vi "Send.vi"(8 "error in (no error)":errorcluster, 10 "Message":refnum<class "BaseMessage.lvclass">, 11 "QueueReader in":refnum<class "MultiQueueReader.lvclass">) -> (0 "error out":errorcluster, 2 "Sent Message":refnum<class "BaseMessage.lvclass">, 3 "QueueReader out":refnum<class "MultiQueueReader.lvclass">)   [LabVIEW 2025, in "MultiQueueReader.lvclass"]
doc: "Send a message to the remote destination"
uses:
  MultiQueueReader.lvclass
  Message/BaseMessage/BaseMessage.lvclass
  MultiQueueReader.lvclass/MultiQueueReader.ctl
  BaseReader/BaseReader.lvclass
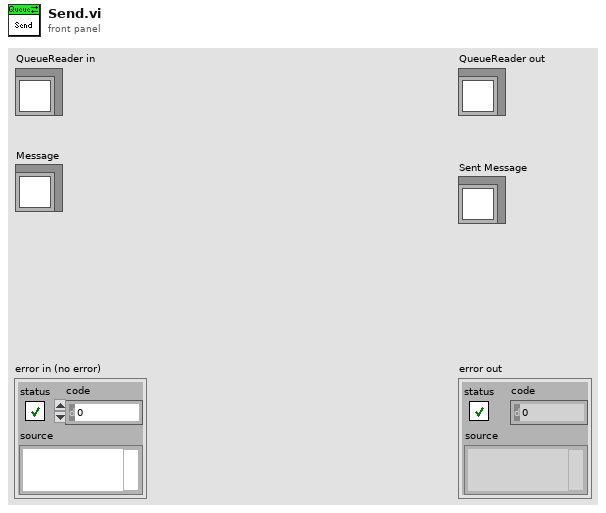
[diagram p1: front panel]
types:
  T1 = typedef "message_queue.ctl" = refnum<queue>
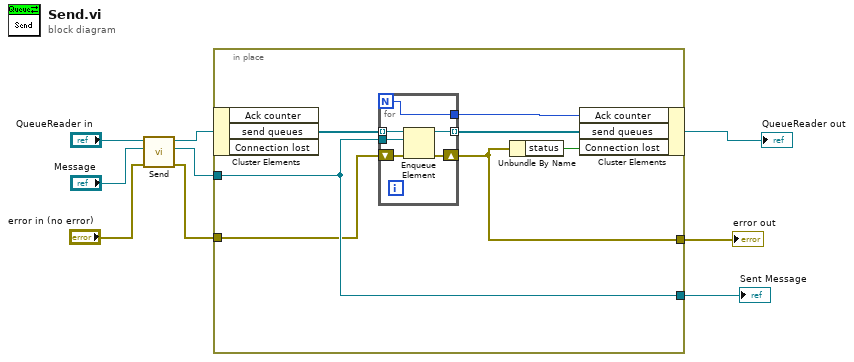
[diagram p0: block diagram]
diagram:
  n1 = call-parent "Send.vi"("error in (no error)"="error in (no error)", "Message"="Message", "BaseReader in"="QueueReader in") -> ("error out"=w1:errorcluster, "Sent Message"=w3:refnum<class "BaseMessage.lvclass">, "BaseReader out"=w5:refnum<class "MultiQueueReader.lvclass">)  [unwired: 6 in]
  n2 = in-place "In Place Element Structure" {
    in-place-border: w3 -> [w16]
    in-place-border: [w16] -> w9
    in-place-border: w1 -> [w14]
    in-place-border: [w12] -> w7
    n3 = in-place-cluster #1(w5) -> ("send queues"=w11:T1[])  [unwired: 2 out]
    n4 = for {
      N -> [w17]
      tunnel: w16 -> [w22]
      tunnel: [w21] -> w15 mode=indexing
      tunnel: w11 -> [w18] mode=indexing
      shift-right: [w19] -> w12
      shift-left: w14 -> [w20]
      tunnel: [w17] -> w10
      n5 = Enqueue Element(queue=w18, element=w22, error in (no error)=w20) -> (queue out=w21:T1, error out=w19:errorcluster)  [unwired: 1 in, 1 out]
    }
    n6 = Unbundle By Name(w12) -> ("status"=w13:bool)
    n7 = in-place-cluster #1("Ack counter"=w10, "send queues"=w15, "Connection lost"=w13) -> (→"QueueReader out":refnum<class "MultiQueueReader.lvclass">)
  }
  "error out" <- w7
  "Sent Message" <- w9
